vi "FTW-CSV-Variant-Headers.vi"(0 "Variant":variant, 1 "Delimiter":string=",", 9 "String Quotes":bool, 11 "error in":errorcluster, 14 "Line Ending":string="\n") -> (4 "CSV String":string, 15 "error out":errorcluster)   [LabVIEW 2015]
uses:
  FTW-CSV-SerializeOptions.ctl
  <vilib>/Utility/Data Type/NI_Data Type.lvlib
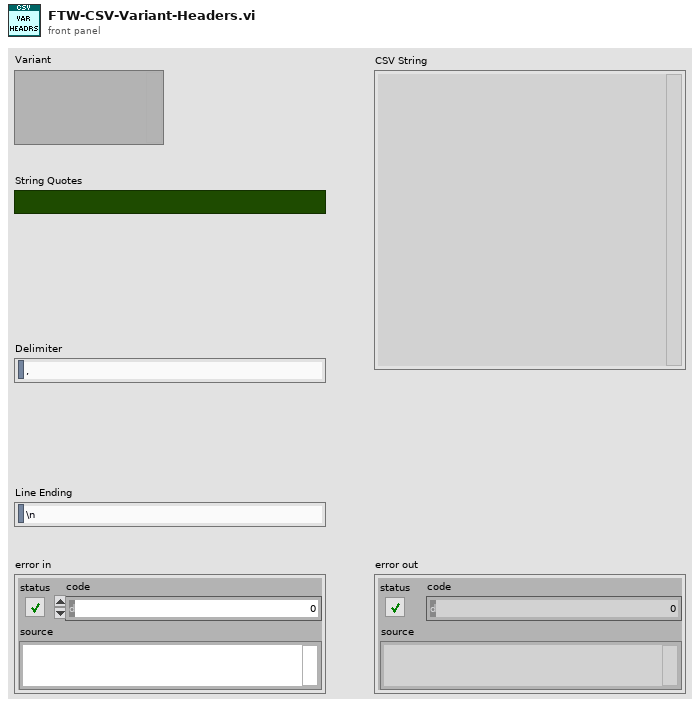
[diagram p1: front panel]
types:
  T1 = typedef "FTW-CSV-SerializeOptions.ctl" = cluster{"String Quotes":bool, "Real Format":string, "Timestamp Format":string, "Delimiter":string}
  T2 = typedef "NI_Data Type.lvlib/Data Type.ctl" = enum8{"Invalid Type", "Void", "I8", "I16", "I32", "I64", "U8", "U16", "U32", "U64", "Single Float", "Double Float", "Extended Float", "Single Complex", "Double Complex", "Extended Complex", "Enum U8", "Enum U16", "Enum U32", "Enum U64", "Single Float With Unit", "Double Float With Unit", "Extended Float With Unit", "Single Complex with Unit", "Double Complex with Unit", "Extended Complex with Unit", "Boolean", "String", "Path", "Picture", "Tag", "Array", "Cluster", "Variant", "LV Variant", "Waveform", "Timestamp", "Digital Waveform", "Digital Data", "ExpressData", "Refnum", "External Data", "VI", "Poly VI", "LabVIEW Class Instance", "Fixed Point"}
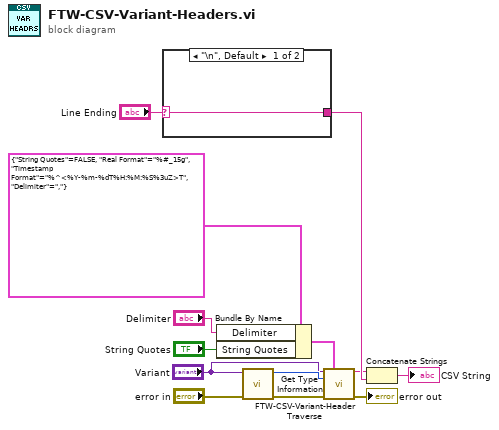
[diagram p0: block diagram]
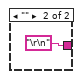
[diagram p2: hidden frame]
diagram:
  n1 = case shown="\"\\n\", Default" "Line Ending" {
    selector: "Line Ending" -> [w14 _]
    tunnel: [w14 "\r\n"] -> w2
    frame "\n", Default {
    }
    frame "" {
    }
  }
  n2 = Bundle By Name(cluster=T1 {"String Quotes"=FALSE, "Real Format"="%#_15g", "Timestamp Format"="%^<%Y-%m-%dT%H:%M:%S%3uZ>T", "Delimiter"=","} ("Options"), "Delimiter"="Delimiter", "String Quotes"="String Quotes") -> (w11:T1)
  n3 = call <vilib>:"Get Type Information.vi"("error in (no error)"="error in", "Variant"="Variant") -> ("error out"=w9:errorcluster, "Type"=w8:T2)  [unwired: 5 in, 3 out]
  n4 = call "FTW-CSV-Variant-HeaderTraverse.vi"("Variant"="Variant", "Options"=w11, "Type"=w8, "error in"=w9) -> ("CSV String"=w1:string, "error out"=→"error out":errorcluster)  [unwired: 10 in]
  n5 = Concatenate Strings(w1, w2) -> (→"CSV String":string)
